vi "Read Sweep Control.json.vi"(8 "error in (no error)":errorcluster, 10 "file (use dialog)":path, 11 "SweepControl in":refnum<class "SweepControl.lvclass">) -> (0 "error out":errorcluster, 2 "data":T1 {"Lockin"."Channels: Lockin"."order" min=1; "Lockin"."Channels: Lockin"."TC (s)" min=1e-05 format="%#_3p"; "Lockin"."Channels: Lockin"."Phase (°)" format="%.3g"; "Lockin"."Channels: Lockin"."f (Hz)" format="%.3g"; "Lockin"."Channels: AO"."f (Hz)" min=0.001 max=10000.0 format="%.3g"; "Lockin"."Channels: AO"."Phase (°)" format="%.3g"; "Lockin"."Channels: AO"."DC (V)" format="%.3p"; "Lockin"."Channels: AO"."Amp (V)" min=0.0 max=10.0 format="%.3p"; "Sweep Control"."Scan parameters"."Rate" format="%.2f"; "Sweep Control"."Scan parameters"."Step" format="%#_6p"; "Sweep Control"."Scan parameters"."End" format="%#_6p"; "Sweep Control"."Scan parameters"."Start" format="%#_6p"}, 3 "SweepControl out":refnum<class "SweepControl.lvclass">)   [LabVIEW 2016, in "SweepControl.lvclass"]
uses:
  SweepControl.lvclass
  Typedefs/Sweep Control Configuration--Cluster.ctl
  Typedefs/Enum - Experiments.ctl
  Typedefs/ScanParamters.ctl
  Typedefs/Cluster - ScanParamters.ctl
  Typedefs/ScanControl.ctl
  Typedefs/Cluster - ScanControl.ctl
  Typedefs/Enum - Priority.ctl
  Typedefs/Enum - Action.ctl
  Control Experiment/Typedefs/Experiment Description--cluster.ctl
  Control Experiment/Typedefs/Instrument--enum.ctl
  Control Experiment/Typedefs/Wiring Description--cluster.ctl
  <userlib>/LevyLab/Lockin-Multichannel/LockinDAQ/Typedefs/AO-cluster.ctl
  <userlib>/LevyLab/Lockin-Multichannel/LockinDAQ/Typedefs/Function-enum.ctl
  <userlib>/LevyLab/Lockin-Multichannel/LockinDAQ/Typedefs/REF-cluster.ctl
  <userlib>/LevyLab/Krohn Hite 7008/typedefs/KH_control_array.ctl
  <userlib>/LevyLab/Krohn Hite 7008/typedefs/KH_control.ctl
  <userlib>/LevyLab/Krohn Hite 7008/typedefs/Channel-Enum.ctl
  <userlib>/LevyLab/Krohn Hite 7008/typedefs/Gain-Enum.ctl
  <userlib>/LevyLab/Krohn Hite 7008/typedefs/Shunt-Enum.ctl
  <userlib>/LevyLab/Krohn Hite 7008/typedefs/Input Configuration-Enum.ctl
  <vilib>/addons/_JKI.lib/Serialization/JSON/JKI JSON Serialization.lvlib
  <userlib>/LevyLab/Krohn Hite 7008/Instrument.KH7008.lvclass
  <userlib>/LevyLab/Lockin-Multichannel/LockinDAQ/LockinDAQ.lvclass
  Control Experiment/Control Experiment.lvclass
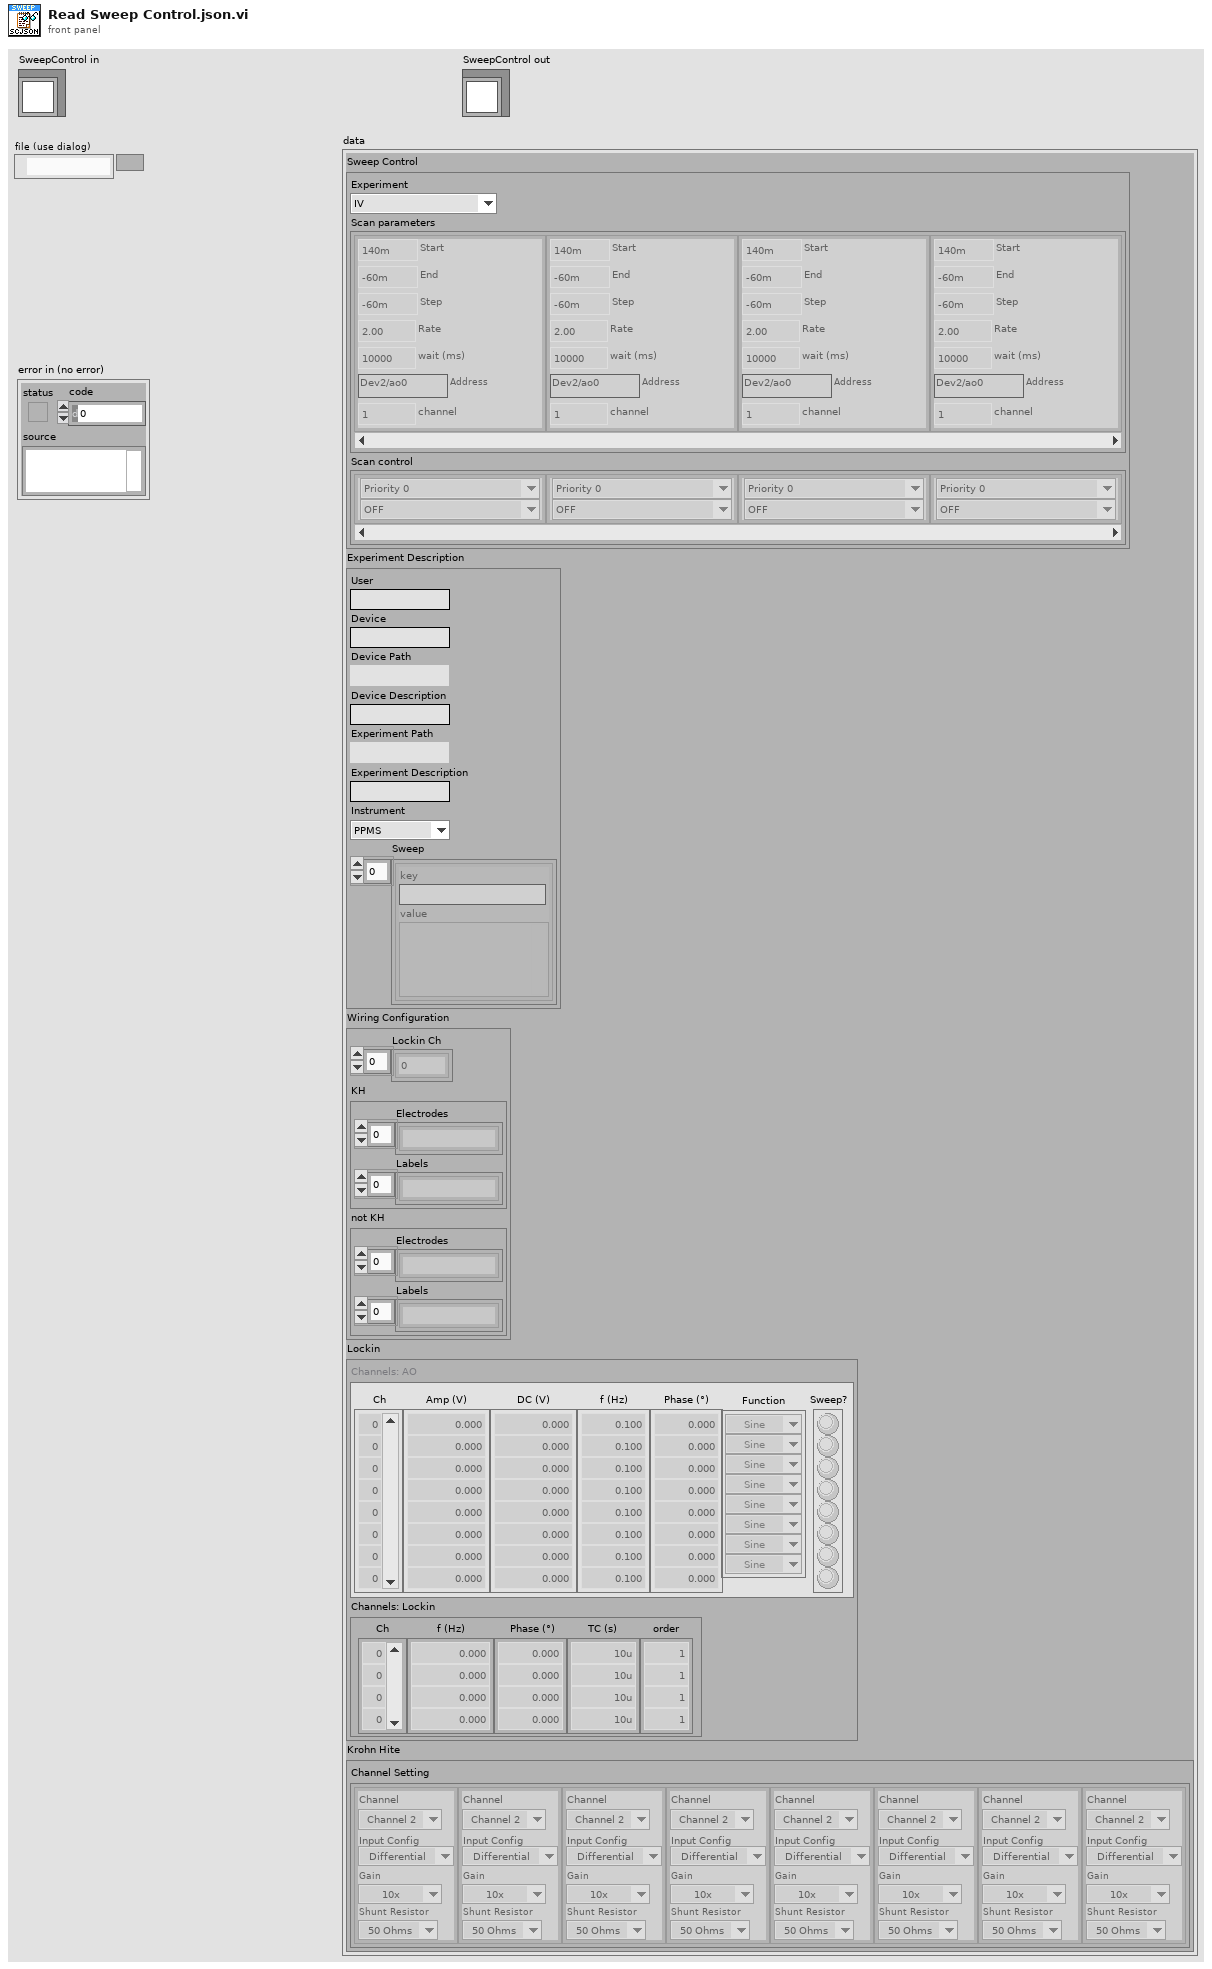
[diagram p1: front panel]
types:
  T1 = typedef "SweepControl.lvclass/Sweep Control Configuration--Cluster.ctl" = cluster{"Sweep Control":cluster{"Experiment":T2, "Scan parameters":T3, "Scan control":T5}, "Experiment Description":T9, "Wiring Configuration":T11, "Lockin":cluster{"Channels: AO":T12, "Channels: Lockin":T14}, "Krohn Hite":cluster{"Channel Setting":T15}}
  T2 = typedef "SweepControl.lvclass/Enum - Experiments.ctl" = enum16{"IV", "Lockin Vsg", "Lockin Sweep", "Lockin time", "AI WFM time", "Lockin (experimental)"}
  T3 = typedef "SweepControl.lvclass/ScanParamters.ctl" = T4[]
  T4 = typedef "SweepControl.lvclass/Cluster - ScanParamters.ctl" = cluster{"Start":dbl, "End":dbl, "Step":dbl, "Rate":dbl, "wait (ms)":u32, "Address":string, "channel":i32}
  T5 = typedef "SweepControl.lvclass/ScanControl.ctl" = T6[]
  T6 = typedef "SweepControl.lvclass/Cluster - ScanControl.ctl" = cluster{"Priority":T7, "Scan name":T8}
  T7 = typedef "SweepControl.lvclass/Enum - Priority.ctl" = enum16{"Priority 0", "Priority 1", "Priority 2", "Priority 3", "Priority 4", "Priority 5"}
  T8 = typedef "SweepControl.lvclass/Enum - Action.ctl" = enum16{"OFF", "DSA_Vamp", "DSA_freq", "DSA_Vsg1", "DSA_Vsg2", "DSA_Vsg3", "DAQ_Vbg", "B_Field", "Humidity", "Temp", "MW_freq1", "MW_freq2", "MW_amplitude1", "MW_amplitude2"}
  T9 = typedef "Control Experiment.lvclass/Experiment Description--cluster.ctl" = cluster{"User":string, "Device":string, "Device Path":path, "Device Description":string, "Experiment Path":path, "Experiment Description":string, "Instrument":T10, "Sweep":cluster{"key":string, "value":variant}[]}
  T10 = typedef "Control Experiment.lvclass/Instrument--enum.ctl" = enum16{"PPMS", "PPMS2", "MFP3D", "CYPHER", "THz1", "THz2", "MNK", "CF900", "JEOL", "AGILENT", "EBL"}
  T11 = typedef "Control Experiment.lvclass/Wiring Description--cluster.ctl" = cluster{"Lockin Ch":i32[], "KH":cluster{"Electrodes":string[], "Labels":string[]}, "not KH":cluster{"Electrodes":string[], "Labels":string[]}}
  T12 = typedef "LockinDAQ.lvclass/AO-cluster.ctl" = cluster{"Ch":i32[], "Amp (V)":dbl[], "DC (V)":dbl[], "f (Hz)":dbl[], "Phase (°)":dbl[], "Function":T13[], "Sweep?":bool[]}
  T13 = typedef "LockinDAQ.lvclass/Function-enum.ctl" = enum16{"Sine", "Triangle", "Square", "Sawtooth"}
  T14 = typedef "LockinDAQ.lvclass/REF-cluster.ctl" = cluster{"Ch":i32[], " f (Hz)":dbl[], "Phase (°)":dbl[], "TC (s)":dbl[], "order":i32[]}
  T15 = typedef "Instrument.KH7008.lvclass/KH_control_array.ctl" = T16[]
  T16 = typedef "Instrument.KH7008.lvclass/KH_control.ctl" = cluster{"Channel":T17, "Gain":T18, "Shunt Resistor":T19, "Input Config":T20}
  T17 = typedef "Instrument.KH7008.lvclass/Channel-Enum.ctl" = enum16{"Channel 1", "Channel 2", "Channel 3", "Channel 4", "Channel 5", "Channel 6", "Channel 7", "Channel 8"}
  T18 = typedef "Instrument.KH7008.lvclass/Gain-Enum.ctl" = enum16{"1x", "10x", "100x", "1000x"}
  T19 = typedef "Instrument.KH7008.lvclass/Shunt-Enum.ctl" = enum16{"Open", "50 Ohms", "500 Ohms", "5k Ohms", "50k Ohms"}
  T20 = typedef "Instrument.KH7008.lvclass/Input Configuration-Enum.ctl" = enum16{"Ground", "SE+ (-gnd)", "SE- (+gnd)", "Differential"}
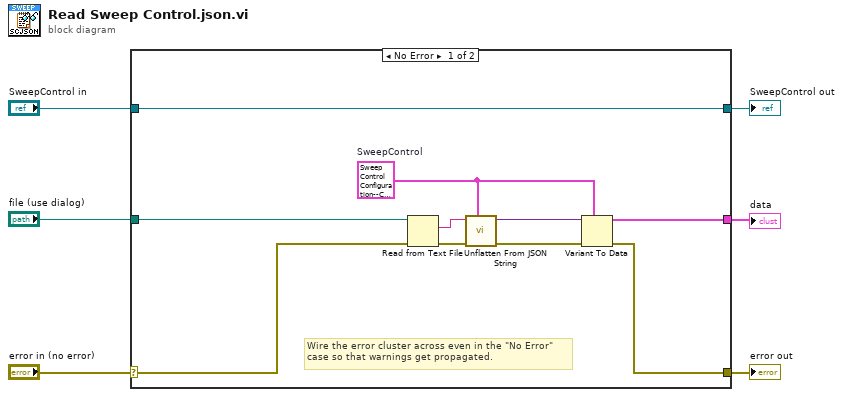
[diagram p0: block diagram]
diagram:
  n1 = case shown="No Error" "error in (no error)" {
    selector: "error in (no error)" -> [w13 w18]
    tunnel: [w11 w18] -> w5
    tunnel: [w16 w17] -> w3
    tunnel: "SweepControl in" -> [w16 w17]
    tunnel: "file (use dialog)" -> [w8 _]
    tunnel: [w7 _] -> w1
    frame No Error {
      w9 = T1 {"Sweep Control"={"Experiment"=enum."IV", "Scan parameters"=[], "Scan control"=[]}, "Experiment Description"={"User"="", "Device"="", "Device Path"=path "", "Device Description"="", "Experiment Path"=path "", "Experiment Description"="", "Instrument"=enum."PPMS", "Sweep"=[]}, "Wiring Configuration"={"Lockin Ch"=[], "KH"={"Electrodes"=[], "Labels"=[]}, "not KH"={"Electrodes"=[], "Labels"=[]}}, "Lockin"={"Channels: AO"={"Ch"=[], "Amp (V)"=[], "DC (V)"=[], "f (Hz)"=[], "Phase (°)"=[], "Function"=[], "Sweep?"=[]}, "Channels: Lockin"={"Ch"=[], " f (Hz)"=[], "Phase (°)"=[], "TC (s)"=[], "order"=[]}}, "Krohn Hite"={"Channel Setting"=[]}}  # SweepControl
      # "Wire the error cluster across even in the \"No Error\"\ncase so that warnings get propagated."
      n2 = Read from Text File(file (use dialog)=w8, error in=w13) -> (text=w14:string, error out=w15:errorcluster)  [unwired: 2 in, 2 out]
      n3 = call <vilib>:"Unflatten From JSON String.vi"("Type and Defaults"=w9, "error in (no error)"=w15, "JSON String"=w14) -> ("error out"=w12:errorcluster, "Variant"=w10:variant)  [unwired: 7 in]
      n4 = Variant To Data(error in=w12, type=w9, Variant=w10) -> (data=w7:T1, error out=w11:errorcluster)
    }
    frame Error {
    }
  }
  "error out" <- w5
  "SweepControl out" <- w3
  "data" <- w1
